vi "Enable Disable.vi"(8 "Error In":errorcluster, 10 "Enable (T)":bool=TRUE, 11 "Timer Handle":T1) -> (0 "Error Out":errorcluster, 3 "Timer Handle":T1)   [LabVIEW 2021, in "Timer-API.lvlib" / "Timer Session.lvclass"]
doc: "This method allows to enable or disable the timer. This effectively means the timer is either paused or running.\n\nYou can specify the input as timer name or timer reference. Using reference executes faster."
uses:
  Timer Session.lvclass
  Timer Session.lvclass/Timer Session.ctl
  Typedefs/Session Handle.ctl
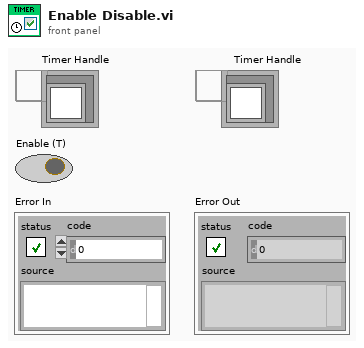
[diagram p1: front panel]
types:
  T1 = typedef "Timer-API.lvlib/Timer Session.lvclass/Session Handle.ctl" = refnum<data-value>
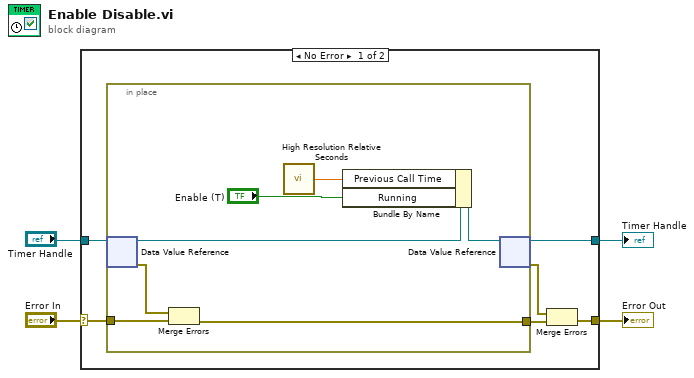
[diagram p0: block diagram]
diagram:
  n1 = case shown="No Error" "Error In" {
    selector: "Error In" -> [w8 w19]
    tunnel: "Timer Handle" -> [w10 w18]
    tunnel: [w5 w19] -> w1
    tunnel: [w9 w18] -> w2
    frame No Error {
      n2 = in-place {
        in-place-border: w8 -> [w15]
        in-place-border: [w13] -> w7
        n3 = in-place-dvr #1(w10) -> (w17:refnum<class "Timer Session.lvclass">, w14:errorcluster)
        n4 = Merge Errors(w14, w15) -> (w13:errorcluster)
        n5 = call <vilib>:"High Resolution Relative Seconds.vi"() -> ("relative seconds"=w12:dbl)
        n6 = Bundle By Name(cluster=w17, "Previous Call Time"=w12, "Running"="Enable (T)") -> (w16:refnum<class "Timer Session.lvclass">)
        n7 = in-place-dvr #1(w16) -> (w9:T1, w6:errorcluster)
      }
      n8 = Merge Errors(w6, w7) -> (w5:errorcluster)
    }
    frame Error {
    }
  }
  "Timer Handle" <- w2
  "Error Out" <- w1
